vi "Event MessengerM Channel Wire  -  Specify Receiving Event Handler.vi"() -> ()   [LabVIEW 2020]
doc: "This example shows how to specify the receiving event structure on the same Event MessengerM Channel connecting those."
uses:
  <extravilib>/ChannelInstances/Event Messenger-dbl.lvlib
  3ea238a4-802d-40cb-9bc8-21683f02d229.vi
  b0398016-5e04-49fd-ad06-9d04750778b2.vi
  1936a7ad-1147-4a36-87f5-8fe3e66ea461.vi
  4618a18b-6ae5-42de-ab17-2c4c956c90ee.vi
  eebb98b5-d8ad-4e6c-a686-31b4d2a186c1.vi
  b1f63473-2a17-44bb-bd61-fec0fcd5c7bc.vi
  82d8d565-bb11-4528-8c4f-ce23458dbc8f.vi
  8cb9dd96-c646-4f19-b11e-f21efaff9273.vi
panel:
  out "Result":dbl
  in  "Max Button":bool
  in  "Multiply Button":bool
  in  "Add Button":bool
  in  "Elements":dbl[](array[numeric])
  in  "Abort Button":bool
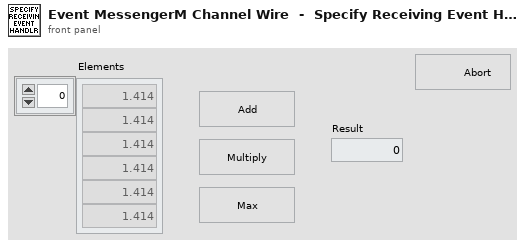
[diagram p1: front panel]
types:
  T1 = typedef "Event MessengerM-a[.](dbl).lvlib/))Channel.ctl" = refnum<queue>
  T2 = typedef "Event Messenger-dbl.lvlib/))Channel.ctl" = refnum<queue>
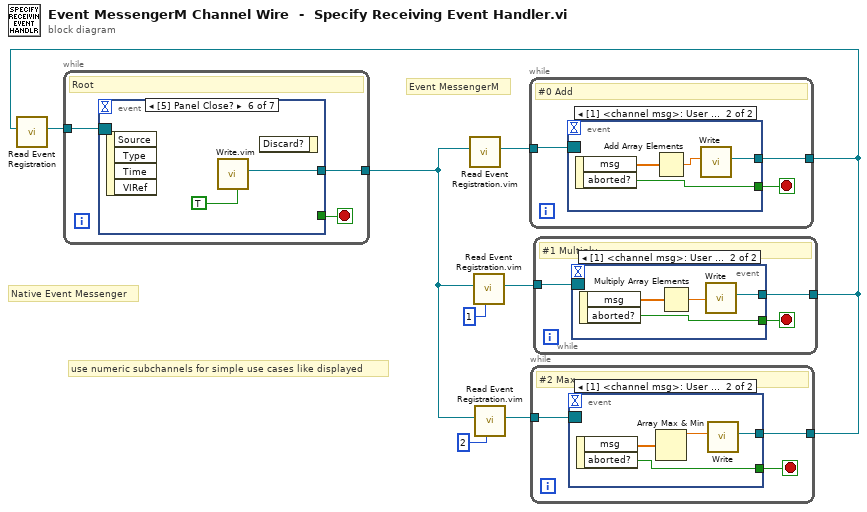
[diagram p0: block diagram]
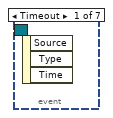
[diagram p2: hidden frame]
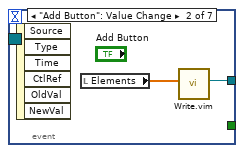
[diagram p3: hidden frame]
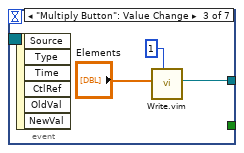
[diagram p4: hidden frame]
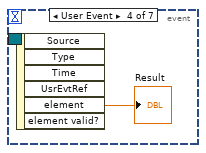
[diagram p5: hidden frame]
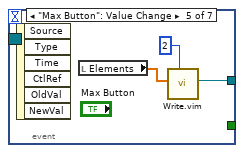
[diagram p6: hidden frame]
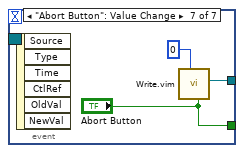
[diagram p7: hidden frame]
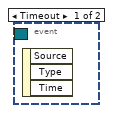
[diagram p8: hidden frame]
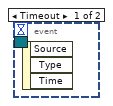
[diagram p9: hidden frame]
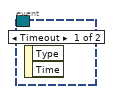
[diagram p10: hidden frame]
diagram:
  # "use numeric subchannels for simple use cases like displayed"
  # "Native Event Messenger"
  # "Event MessengerM"
  n1 = call <extravilib>:"Read Event Registration.vi"("channel"=w3) -> ("event registration refnum"=w4:refnum<event-registration>)  [unwired: 10 in]
  n2 = while {
    tunnel: [w10] -> w6
    tunnel: w4 -> [w9]
    stop <- w11 stop-if-true
    # "Root"
    n3 = event shown="[5] Panel Close?" {
      selector: w9 -> [_ _ _ _ _ _ _]
      dyn-events: _ -> [_ _ _ _ _ _ _]
      timeout: _ -> [_ _ _ _ _ _ _]
      tunnel: [_ _ _ _ _ _ "Abort Button"] -> w11
      tunnel: [_ w13 w14 _ w19 w22 w25] -> w10
      event Timeout {
        n4 = event-data() -> ()  [unwired: 1 in, 3 out]
      }
      event "Add Button": Value Change {
        n5 = event-data() -> ()  [unwired: 1 in, 6 out]
        n6 = local read "Elements"() -> (w12:dbl[])
        n7 = call "Write.vim"("element"=w12) -> ("channel"=w13:T1)  [unwired: 9 in, 1 out]
      }
      event "Multiply Button": Value Change {
        n8 = event-data() -> ()  [unwired: 1 in, 6 out]
        n9 = call "Write.vim"("subchannel"=1 ("subchannel (0)"), "element"="Elements") -> ("channel"=w14:T1)  [unwired: 8 in, 1 out]
      }
      event User Event {
        n10 = event-data() -> ("element"=→"Result":dbl)  [unwired: 1 in, 5 out]
      }
      event "Max Button": Value Change {
        n11 = event-data() -> ()  [unwired: 1 in, 6 out]
        n12 = local read "Elements"() -> (w20:dbl[])
        n13 = call "Write.vim"("subchannel"=2 ("subchannel (0)"), "element"=w20) -> ("channel"=w19:T1)  [unwired: 8 in, 1 out]
      }
      event Panel Close? {
        n14 = event-data() -> ()  [unwired: 1 in, 4 out]
        n15 = call "Write.vim"("abort all (F)"=TRUE) -> ("channel"=w22:T1)  [unwired: 9 in, 1 out]
        n16 = event-data() -> ()  [unwired: 2 in, 1 out]
      }
      event "Abort Button": Value Change {
        n17 = event-data() -> ()  [unwired: 1 in, 6 out]
        n18 = call "Write.vim"("abort all (F)"="Abort Button", "subchannel"=0) -> ("channel"=w25:T1)  [unwired: 8 in, 1 out]
      }
    }
  }
  n19 = call "Read Event Registration.vim"("channel"=w6) -> ("event registration refnum"=w8:refnum<event-registration>)  [unwired: 10 in]
  n20 = call "Read Event Registration.vim"("subchannel"=1 ("subchannel (0)"), "channel"=w6) -> ("event registration refnum"=w7:refnum<event-registration>)  [unwired: 9 in]
  n21 = call "Read Event Registration.vim"("subchannel"=2 ("subchannel (0)"), "channel"=w6) -> ("event registration refnum"=w5:refnum<event-registration>)  [unwired: 9 in]
  n22 = while {
    tunnel: w8 -> [w28]
    tunnel: [w26] -> w3
    stop <- w27 stop-if-true
    # "#0 Add"
    n23 = event shown="[1] <channel msg>: User Event" {
      selector: w28 -> [_ _]
      dyn-events: _ -> [_ _]
      timeout: _ -> [_ _]
      tunnel: [_ w32] -> w27
      tunnel: [_ w29] -> w26
      event Timeout {
        n24 = event-data() -> ()  [unwired: 1 in, 2 out]
      }
      event User Event {
        n25 = event-data() -> ("msg"=w31:dbl[], "aborted?"=w32:bool)  [unwired: 1 in]
        n26 = Add Array Elements(numeric array=w31) -> (sum=w30:dbl)
        n27 = call <extravilib>:"Write.vi"("element"=w30) -> ("channel"=w29:T2)  [unwired: 9 in, 1 out]
      }
    }
  }
  n28 = while {
    tunnel: w5 -> [w35]
    tunnel: w3 -> [w34]
    stop <- w33 stop-if-true
    # "#2 Max"
    n29 = event shown="[1] <channel msg>: User Event" {
      selector: w35 -> [_ _]
      dyn-events: _ -> [_ _]
      timeout: _ -> [_ _]
      tunnel: [_ w37] -> w34
      tunnel: [_ w36] -> w33
      event Timeout {
        n30 = event-data() -> ()  [unwired: 1 in, 3 out]
      }
      event User Event {
        n31 = event-data() -> ("msg"=w39:dbl[], "aborted?"=w36:bool)  [unwired: 1 in]
        n32 = Array Max & Min(array=w39) -> (max value=w38:dbl)  [unwired: 3 out]
        n33 = call <extravilib>:"Write.vi"("element"=w38) -> ("channel"=w37:T2)  [unwired: 9 in, 1 out]
      }
    }
  }
  n34 = while {
    tunnel: w7 -> [w42]
    tunnel: w3 -> [w40]
    stop <- w41 stop-if-true
    # "#1 Multiply"
    n35 = event shown="[1] <channel msg>: User Event" {
      selector: w42 -> [_ _]
      dyn-events: _ -> [_ _]
      timeout: _ -> [_ _]
      tunnel: [_ w46] -> w41
      tunnel: [_ w43] -> w40
      event Timeout {
        n36 = event-data() -> ()  [unwired: 1 in, 3 out]
      }
      event User Event {
        n37 = event-data() -> ("msg"=w45:dbl[], "aborted?"=w46:bool)  [unwired: 1 in]
        n38 = Multiply Array Elements(1:w45) -> (0:w44:dbl)
        n39 = call <extravilib>:"Write.vi"("element"=w44) -> ("channel"=w43:T2)  [unwired: 9 in, 1 out]
      }
    }
  }
